vi "gpib.vi"() -> ()   [LabVIEW 2023]
panel:
  out "error out":errorcluster
  in  "Cutoff current":dbl
  in  "curr set":dbl(knob) min=-5.0 max=5.0 scale=0.0..5.0
  in  "volt set":dbl(knob) min=-20.0 max=20.0 step=0.0001 scale=0.0..20.0
  out "output current":dbl
  out "output voltage":dbl
  out "Current":dbl(graph)
  out "Voltage":dbl(graph)
  in  "output off/on":bool
  in  "stop":bool
  in  "Instrument address":string="2"
  in  "byte count 2":i32
  out "curr output":string
  in  "byte count":i32
  out "Volt output":string
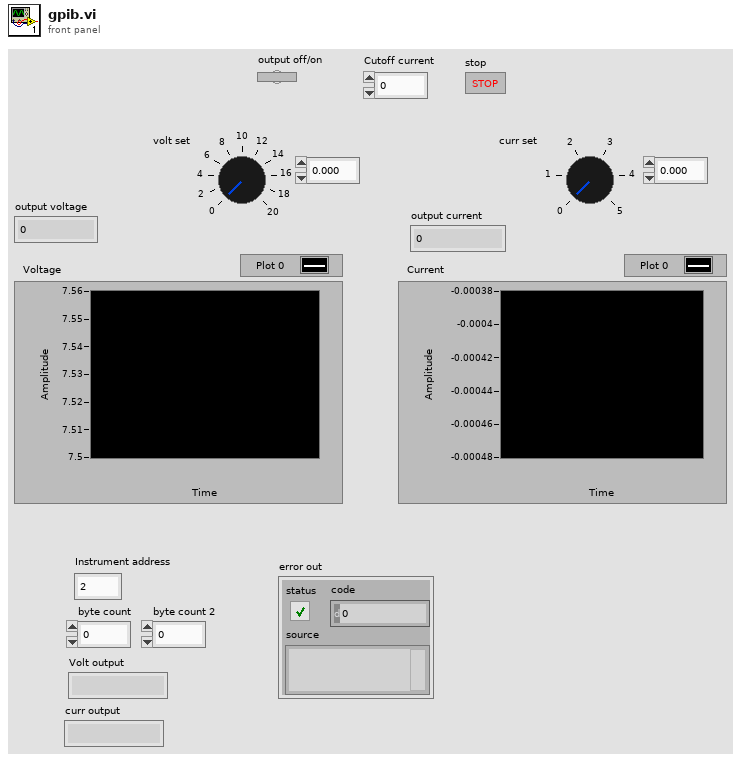
[diagram p1: front panel]
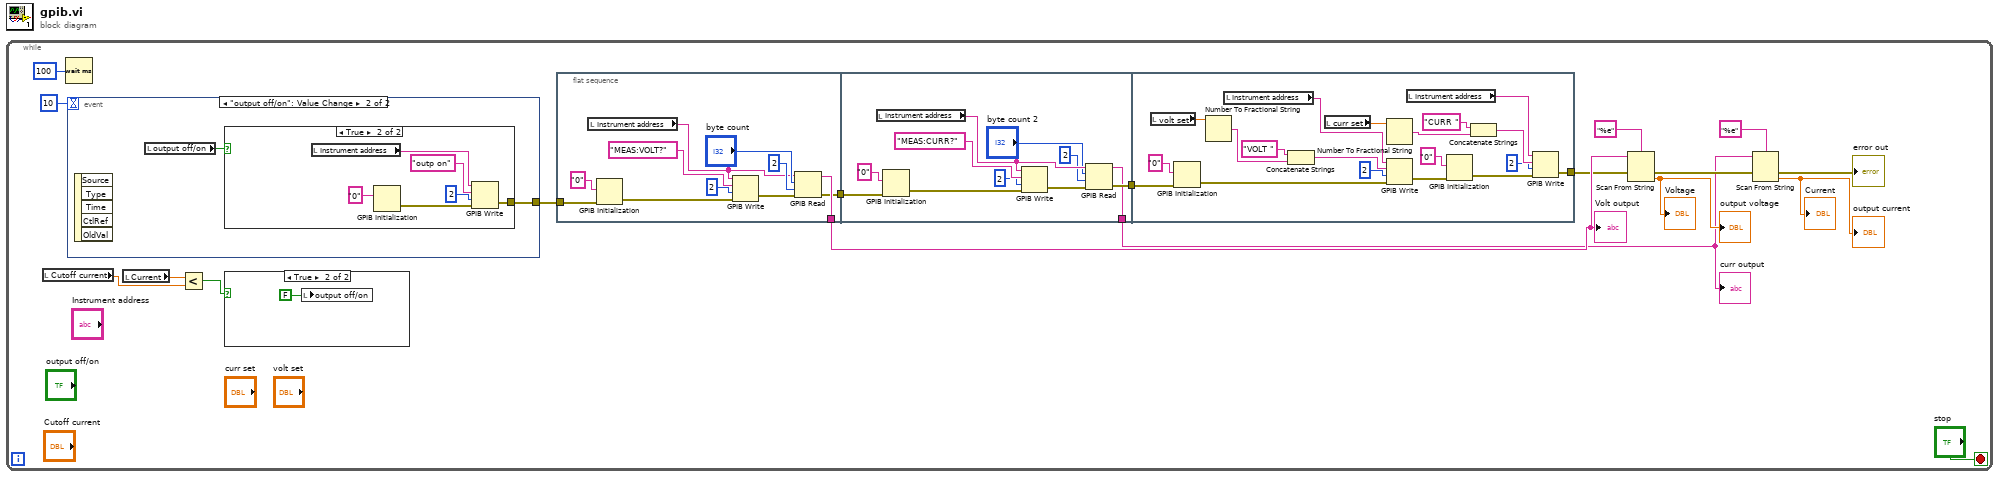
[diagram p0: block diagram]
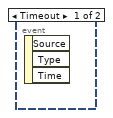
[diagram p3: hidden frame]
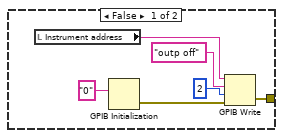
[diagram p4: hidden frame]
diagram:
  n1 = while {
    stop <- "stop" stop-if-true
    n2 = local read "Cutoff current"() -> (w8:dbl)
    n3 = Wait (ms)(milliseconds to wait=u32 100) -> ()  [unwired: 1 out]
    n4 = event shown="[1] \"output off/on\": Value Change" {
      selector: _ -> [_ _]
      dyn-events: _ -> [_ _]
      timeout: 10 -> [_ _]
      tunnel: [_ w61] -> w1
      event Timeout {
        n5 = event-data() -> ()  [unwired: 1 in, 3 out]
      }
      event "output off/on": Value Change {
        n6 = event-data() -> ()  [unwired: 1 in, 5 out]
        n7 = local read "output off/on"() -> (w62:bool)
        n8 = case shown="True" w62 {
          tunnel: [w63 w69] -> w61
          frame False {
            n9 = local read "Instrument address"() -> (w64:string)
            n10 = GPIB Initialization(6:"0" ("address string")) -> (0:w68:errorcluster)  [unwired: 6 in]
            n11 = GPIB Write(0:w64, 1:"outp off" ("data"), 2:i16 2 ("mode (0)"), 3:w68) -> (6:w63:errorcluster)  [unwired: 1 in, 1 out]
          }
          frame True {
            n12 = local read "Instrument address"() -> (w74:string)
            n13 = GPIB Initialization(6:"0" ("address string")) -> (0:w73:errorcluster)  [unwired: 6 in]
            n14 = GPIB Write(0:w74, 1:"outp on" ("data"), 2:i16 2 ("mode (0)"), 3:w73) -> (6:w69:errorcluster)  [unwired: 1 in, 1 out]
          }
        }
      }
    }
    n15 = local read "Current"() -> (w10:dbl)
    n16 = Less?(x=w10, y=w8) -> (x < y?=w9:bool)
    n17 = case shown="True" w9 {
      frame False {
      }
      frame True {
        n18 = local write "output off/on"(FALSE) -> ()
      }
    }
    n19 = flat-sequence {
      tunnel: [w21] -> w6
      tunnel: [w20] -> w7
      tunnel: w1 -> [w19]
      tunnel: w7 -> [w32]
      tunnel: [w31] -> w5
      tunnel: [w30] -> w4
      tunnel: w5 -> [w43]
      tunnel: [w41] -> w3
      frame #0 {
        n20 = local read "Instrument address"() -> (w23:string)
        n21 = GPIB Initialization(4:w19, 6:"0" ("address string")) -> (0:w29:errorcluster)  [unwired: 5 in]
        n22 = GPIB Write(0:w23, 1:"MEAS:VOLT?" ("data"), 2:i16 2 ("mode (0)"), 3:w29) -> (6:w26:errorcluster)  [unwired: 1 in, 1 out]
        n23 = GPIB Read(0:w23, 1:"byte count", 2:i16 2 ("mode (0)"), 3:w26) -> (5:w21:string, 7:w20:errorcluster)  [unwired: 1 in, 1 out]
      }
      frame #1 {
        n24 = local read "Instrument address"() -> (w40:string)
        n25 = GPIB Initialization(4:w32, 6:"0" ("address string")) -> (0:w37:errorcluster)  [unwired: 5 in]
        n26 = GPIB Write(0:w40, 1:"MEAS:CURR?" ("data"), 2:i16 2 ("mode (0)"), 3:w37) -> (6:w38:errorcluster)  [unwired: 1 in, 1 out]
        n27 = GPIB Read(0:w40, 1:"byte count 2", 2:i16 2 ("mode (0)"), 3:w38) -> (5:w30:string, 7:w31:errorcluster)  [unwired: 1 in, 1 out]
      }
      frame #2 {
        n28 = local read "volt set"() -> (w58:dbl)
        n29 = GPIB Initialization(4:w43, 6:"0" ("address string")) -> (0:w55:errorcluster)  [unwired: 5 in]
        n30 = Number To Fractional String(number=w58) -> (F-format string=w57:string)  [unwired: 3 in]
        n31 = local read "Instrument address"() -> (w59:string)
        n32 = Concatenate Strings("VOLT " ("data"), w57) -> (w56:string)
        n33 = local read "curr set"() -> (w51:dbl)
        n34 = Number To Fractional String(number=w51) -> (F-format string=w52:string)  [unwired: 3 in]
        n35 = GPIB Write(0:w59, 1:w56, 2:i16 2 ("mode (0)"), 3:w55) -> (6:w42:errorcluster)  [unwired: 1 in, 1 out]
        n36 = local read "Instrument address"() -> (w50:string)
        n37 = GPIB Initialization(4:w42, 6:"0" ("address string")) -> (0:w54:errorcluster)  [unwired: 5 in]
        n38 = Concatenate Strings("CURR " ("data"), w52) -> (w53:string)
        n39 = GPIB Write(0:w50, 1:w53, 2:i16 2 ("mode (0)"), 3:w54) -> (6:w41:errorcluster)  [unwired: 1 in, 1 out]
      }
    }
    n40 = Scan From String(format string="%e", input string=w6, error in=w3) -> (error out=w11:errorcluster, output 1=→"Voltage" →"output voltage":dbl)  [unwired: 2 in, 2 out]
    n41 = Scan From String(format string="%e", input string=w4, error in=w11) -> (error out=→"error out":errorcluster, output 1=→"Current" →"output current":dbl)  [unwired: 2 in, 2 out]
    "Volt output" <- w6
    "curr output" <- w4
  }
